vi "Actor Core.vi"(8 "error in":errorcluster, 11 "DER in":refnum<class "DER.lvclass">) -> (0 "error out":errorcluster, 3 "Actor out":refnum<class "Actor.lvclass">)   [LabVIEW 2018, in "DER Actor.lvlib" / "DER.lvclass"]
doc: "(<B>Filename</B>: Actor Framework.lvlib:Actor.lvclass:Actor Core.vi)\n\nReceives messages to the actor, reacts to them, and initiates any error handling that may shut the actor down.\n\nDescendant classes may override this VI to append parallel tasks for the actor to complete while it handles messages. Overrides use the Call Parent Method node."
uses:
  DER.lvclass
  C:/Users/Administrator/Desktop/2018LabVIEW EMS/EMS Generic Actor/EMS Generic/EMS Generic.lvclass
  <vilib>/ActorFramework/Actor/Actor.lvclass
  EMS Generic Actor/EMS Generic/EMS Generic.lvclass/EMS Generic.ctl
  <vilib>/ORNL/CSEISMIC DDS/CSEISMIC DDS Base/CSEISMIC DDS.lvclass/CSEISMIC DDS.ctl
  <vilib>/ORNL/CSEISMIC DDS/CSEISMIC DDS Base/Accessors/Write DDS Reference.vi
  <vilib>/ORNL/CSEISMIC DDS/CSEISMIC DDS Base/Accessors/Read DDS Reference.vi
  <vilib>/ORNL/CSEISMIC DDS/DDS Reader/DDS Reader.lvclass
  C:/Program Files (x86)/National Instruments/LabVIEW 2018/vi.lib/ORNL/CSEISMIC DDS/CSEISMIC DDS Base/CSEISMIC DDS.lvclass
  <vilib>/ORNL/CSEISMIC DDS/CSEISMIC DDS Base/Error Handler.vi
  Device DDS Communications Framework/Device DDS Communications/Device DDS Communications.lvclass
  EMS Generic Actor/EMS Generic/EMS Generic.lvclass
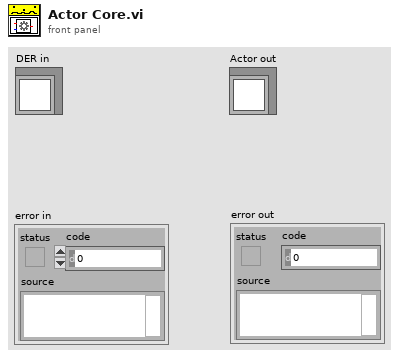
[diagram p1: front panel]
types:
  T1 = typedef "CSEISMIC DDS.lvlib/CSEISMIC DDS.lvclass/DeviceID.ctl" = string
  T2 = typedef "CSEISMIC DDS.lvlib/CSEISMIC DDS.lvclass/DER_Status.ctl" = cluster{"DeviceID":T1, "VFControl":bool, "PControl":bool, "QControl":bool, "PFControl":bool, "PVControl":bool, "Droop":bool, "Unbalanced":bool, "MicrogridVF":bool, "RealDroop(kW)":T3, "ReactiveDroop(kVar)":T3}
  T3 = typedef "CSEISMIC DDS.lvlib/CSEISMIC DDS.lvclass/DroopCurve.ctl" = cluster{"XMin":dbl, "XMax":dbl, "YMin":dbl, "YMax":dbl}
  T4 = typedef "LVDDS_library.lvlib/DDS Sample Info.ctl" = cluster{"DDS_SampleStateKind":enum32{"DDS_INVALID_SAMPLE_STATE", "DDS_READ_SAMPLE_STATE", "DDS_NOT_READ_SAMPLE_STATE"}, "DDS_ViewStateKind":enum32{"DDS_INVALID_SAMPLE_STATE", "DDS_NEW_VIEW_STATE", "DDS_NOT_NEW_VIEW_STATE"}, "DDS_InstanceStateKind":enum32{"DDS_INVALID_STATE", "DDS_ALIVE_INSTANCE_STATE", "DDS_NOT_ALIVE_DISPOSED_INSTANCE_STATE", "", "DDS_NOT_ALIVE_NO_WRITERS_INSTANCE_STATE"}, "sec":i32, "nanosec":u32, "valid_data":bool}
  T5 = typedef "CSEISMIC DDS.lvlib/CSEISMIC DDS.lvclass/DER_Info.ctl" = cluster{"DeviceID":T1, "LineConfig":u8[], "NominalVoltage(V)":dbl, "PowerRating(kVA)":dbl, "VFControl":bool, "PControl":bool, "QControl":bool, "PFControl":bool, "PVControl":bool, "Droop":bool, "DroopConfigurable":bool, "Unbalanced":bool}
  T6 = typedef "CSEISMIC DDS.lvlib/CSEISMIC DDS.lvclass/DER_Measurement.ctl" = cluster{"DeviceID":T1, "Voltage":dbl[], "Current":dbl[], "RealPower":dbl[], "ReactivePower":dbl[], "LineConfig":u8[], "Frequency":dbl}
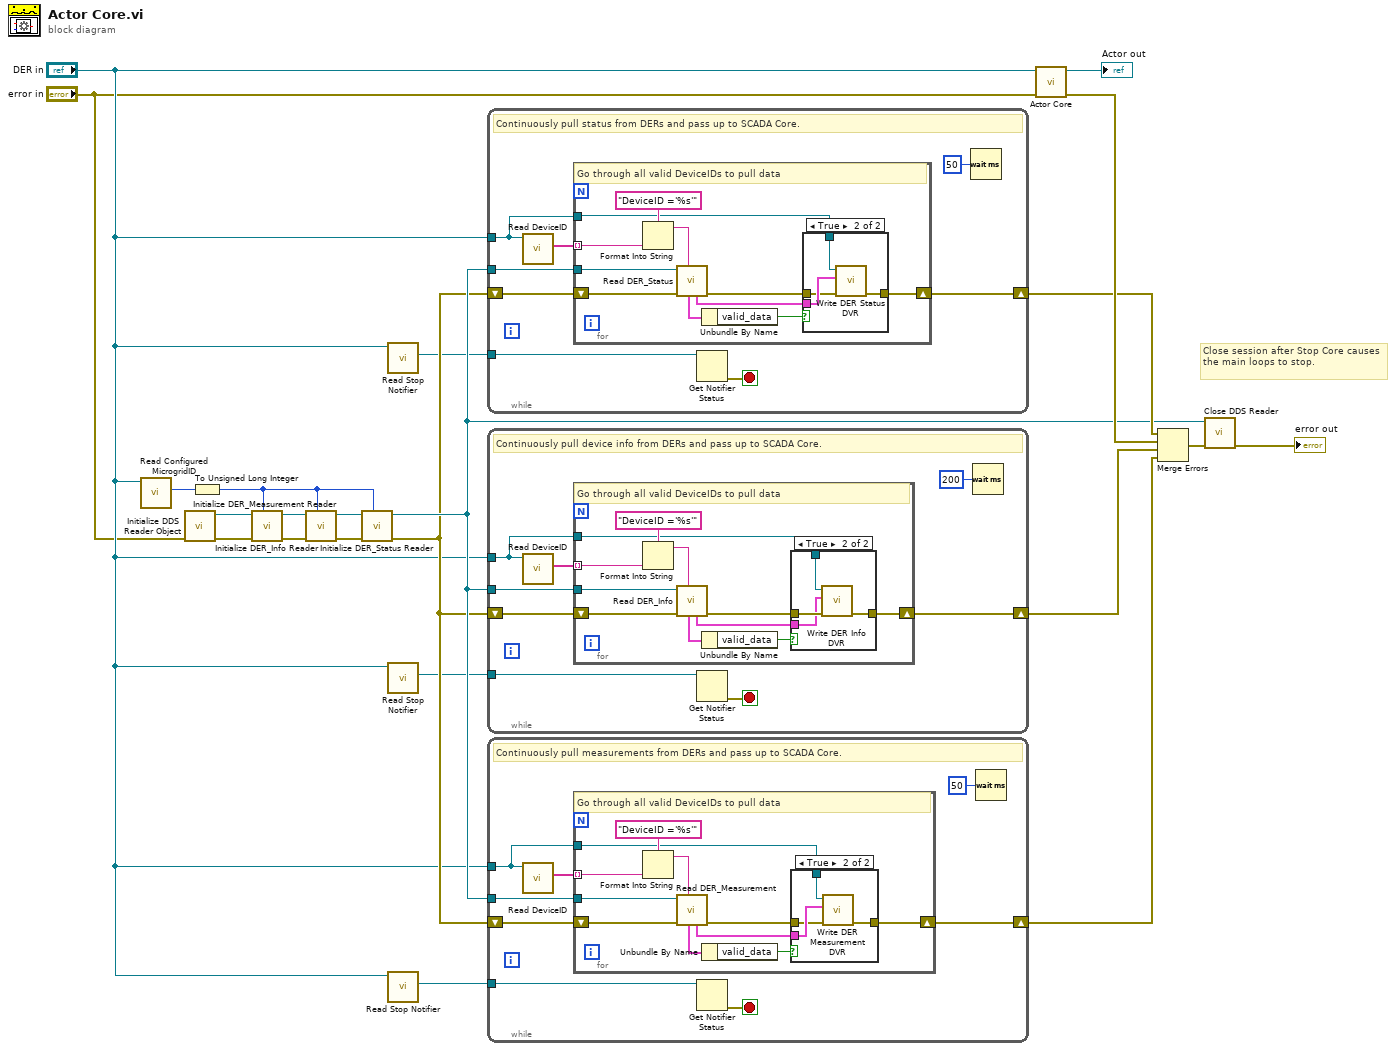
[diagram p0: block diagram]
diagram:
  # "Close session after Stop Core causes the main loops to stop."
  n1 = call "Read Configured MicrogridID.vi"("EMS Generic in"="DER in") -> ("Microgrid ID"=w20:u8)  [unwired: 8 in, 2 out]
  n2 = call <vilib>:"Initialize DDS Reader Object.vi"("error in"="error in") -> ("error out"=w18:errorcluster, "DDS Reader out"=w17:refnum<class "DDS Reader.lvclass">)  [unwired: 9 in]
  n3 = To Unsigned Long Integer(number=w20) -> (unsigned 32bit integer=w3:u32)
  n4 = call <vilib>:"Initialize DER_Info Reader.vi"("MicrogridID"=w3, "error in"=w18, "DDS Reader in"=w17) -> ("error out"=w19:errorcluster, "DDS Reader out"=w16:refnum<class "DDS Reader.lvclass">)  [unwired: 7 in]
  n5 = call <vilib>:"Initialize DER_Measurement Reader.vi"("MicrogridID"=w3, "error in"=w19, "DDS Reader in"=w16) -> ("error out"=w8:errorcluster, "DDS Reader out"=w10:refnum<class "DDS Reader.lvclass">)  [unwired: 7 in]
  n6 = call <vilib>:"Initialize DER_Status Reader.vi"("MicrogridID"=w3, "error in"=w8, "DDS Reader in"=w10) -> ("error out"=w7:errorcluster, "DDS Reader out"=w9:refnum<class "DDS Reader.lvclass">)  [unwired: 7 in]
  n7 = call "Read Stop Notifier.vi"("EMS Generic in"="DER in") -> ("stop"=w4:refnum<notifier>)  [unwired: 9 in, 1 out]
  n8 = call "Read Stop Notifier.vi"("EMS Generic in"="DER in") -> ("stop"=w6:refnum<notifier>)  [unwired: 9 in, 1 out]
  n9 = call "Read Stop Notifier.vi"("EMS Generic in"="DER in") -> ("stop"=w11:refnum<notifier>)  [unwired: 9 in, 1 out]
  n10 = while {
    tunnel: w4 -> [w30]
    shift-right: [w24] -> w14
    shift-left: w7 -> [w26]
    tunnel: "DER in" -> [w23]
    tunnel: w9 -> [w25]
    stop <- w29 stop-if-true
    # "Continuously pull status from DERs and pass up to SCADA Core."
    n11 = call-dynamic "Read DeviceID.vi"("Device DDS Communications in"=w23) -> ("DeviceID"=w27:T1[])  [unwired: 9 in, 1 out]
    n12 = for {
      shift-right: [w32] -> w24
      shift-left: w26 -> [w40]
      tunnel: w27 -> [w38] mode=indexing
      tunnel: w25 -> [w41]
      tunnel: w23 -> [w31]
      # "Go through all valid DeviceIDs to pull data"
      n13 = Format Into String(format string="DeviceID ='%s'", w38) -> (resulting string=w37:string)  [unwired: 2 in, 1 out]
      n14 = call <vilib>:"Read DER_Status.vi"("Query condition"=w37, "error in"=w40, "DDS Reader in"=w41) -> ("error out"=w33:errorcluster, "data"=w34:T2, "DDS Sample Info"=w36:T4)  [unwired: 5 in, 1 out]
      n15 = Unbundle By Name(w36) -> ("valid_data"=w35:bool)
      n16 = case shown="True" w35 {
        tunnel: w34 -> [_ w46]
        tunnel: w33 -> [w42 w45]
        tunnel: [w42 w44] -> w32
        tunnel: w31 -> [_ w43]
        frame False {
        }
        frame True {
          n17 = call "Write DER Status DVR.vi"("error in"=w45, "DER_Status"=w46, "EMS Generic in"=w43) -> ("error out"=w44:errorcluster)  [unwired: 7 in, 1 out]
        }
      }
    }
    n18 = Get Notifier Status(notifier=w30) -> (error out=w29:errorcluster)  [unwired: 1 in, 4 out]
    n19 = Wait (ms)(milliseconds to wait=u32 50) -> ()  [unwired: 1 out]
  }
  n20 = while {
    tunnel: w6 -> [w54]
    shift-right: [w47] -> w13
    shift-left: w7 -> [w50]
    tunnel: "DER in" -> [w48]
    tunnel: w9 -> [w49]
    stop <- w53 stop-if-true
    # "Continuously pull device info from DERs and pass up to SCADA Core."
    n21 = call-dynamic "Read DeviceID.vi"("Device DDS Communications in"=w48) -> ("DeviceID"=w51:T1[])  [unwired: 9 in, 1 out]
    n22 = for {
      shift-right: [w56] -> w47
      shift-left: w50 -> [w64]
      tunnel: w51 -> [w62] mode=indexing
      tunnel: w49 -> [w65]
      tunnel: w48 -> [w55]
      # "Go through all valid DeviceIDs to pull data"
      n23 = Format Into String(format string="DeviceID ='%s'", w62) -> (resulting string=w61:string)  [unwired: 2 in, 1 out]
      n24 = call <vilib>:"Read DER_Info.vi"("Query condition"=w61, "error in"=w64, "DDS Reader in"=w65) -> ("error out"=w57:errorcluster, "data"=w58:T5, "DDS Sample Info"=w60:T4)  [unwired: 5 in, 1 out]
      n25 = Unbundle By Name(w60) -> ("valid_data"=w59:bool)
      n26 = case shown="True" w59 {
        tunnel: [w66 w69] -> w56
        tunnel: w58 -> [_ w68]
        tunnel: w57 -> [w66 w70]
        tunnel: w55 -> [_ w67]
        frame False {
        }
        frame True {
          n27 = call "Write DER Info DVR.vi"("error in"=w70, "DER_Info"=w68, "EMS Generic in"=w67) -> ("error out"=w69:errorcluster)  [unwired: 7 in, 1 out]
        }
      }
    }
    n28 = Get Notifier Status(notifier=w54) -> (error out=w53:errorcluster)  [unwired: 1 in, 4 out]
    n29 = Wait (ms)(milliseconds to wait=u32 200) -> ()  [unwired: 1 out]
  }
  n30 = while {
    tunnel: w11 -> [w78]
    shift-right: [w72] -> w12
    shift-left: w7 -> [w74]
    tunnel: "DER in" -> [w71]
    tunnel: w9 -> [w73]
    stop <- w77 stop-if-true
    # "Continuously pull measurements from DERs and pass up to SCADA Core."
    n31 = call-dynamic "Read DeviceID.vi"("Device DDS Communications in"=w71) -> ("DeviceID"=w75:T1[])  [unwired: 9 in, 1 out]
    n32 = for {
      shift-right: [w80] -> w72
      shift-left: w74 -> [w88]
      tunnel: w75 -> [w86] mode=indexing
      tunnel: w73 -> [w89]
      tunnel: w71 -> [w79]
      # "Go through all valid DeviceIDs to pull data"
      n33 = Format Into String(format string="DeviceID ='%s'", w86) -> (resulting string=w85:string)  [unwired: 2 in, 1 out]
      n34 = call <vilib>:"Read DER_Measurement.vi"("Query condition"=w85, "error in"=w88, "DDS Reader in"=w89) -> ("error out"=w81:errorcluster, "data"=w82:T6, "DDS Sample Info"=w84:T4)  [unwired: 5 in, 1 out]
      n35 = Unbundle By Name(w84) -> ("valid_data"=w83:bool)
      n36 = case shown="True" w83 {
        tunnel: w82 -> [_ w94]
        tunnel: w81 -> [w90 w93]
        tunnel: [w90 w92] -> w80
        tunnel: w79 -> [_ w91]
        frame False {
        }
        frame True {
          n37 = call "Write DER Measurement DVR.vi"("error in"=w93, "DER_Measurement"=w94, "EMS Generic in"=w91) -> ("error out"=w92:errorcluster)  [unwired: 7 in, 1 out]
        }
      }
    }
    n38 = Get Notifier Status(notifier=w78) -> (error out=w77:errorcluster)  [unwired: 1 in, 4 out]
    n39 = Wait (ms)(milliseconds to wait=u32 50) -> ()  [unwired: 1 out]
  }
  n40 = call-parent "Actor Core.vi"("error in"="error in", "Actor in"="DER in") -> ("error out"=w22:errorcluster, "Actor out"=→"Actor out":refnum<class "Actor.lvclass">)  [unwired: 8 in]
  n41 = Merge Errors(w14, w22, w13, w12) -> (w15:errorcluster)
  n42 = call <vilib>:"Close DDS Reader.vi"("error in"=w15, "DDS Reader in"=w9) -> ("error out"=→"error out":errorcluster)  [unwired: 9 in]
